vi "api_mqttSubscribe.vi"(0 "mqtt.lvclass in":refnum<class "mqtt.lvclass">, 5 "subscriptionInfo":T1[](array[typedef])=[{"Topic"="a/b", "QoS"=enum."At least once"}], 9 "messageID":u16=1, 11 "error in (no error)":errorcluster) -> (4 "mqtt.lvclass out":refnum<class "mqtt.lvclass">, 6 "success":bool, 15 "error out":errorcluster)   [LabVIEW 2018, in "labview-mqtt.lvlib" / "mqtt.lvclass"]
uses:
  mqtt.lvclass
  mqttTypedef/mqttSubscribeCluster.ctl
  mqttTypedef/mqttQOSlevel.ctl
  mqttTypedef/mqttMessageType.ctl
  mqttCmd/mqttCmdSubscribe/mqttCmdSubscribe.lvclass
  D:/mqtt-LabVIEW/src/class/mqtt/mqttCmd/mqttCmd.lvclass
  mqttCmd/mqttCmdSubscribe/mqttCmdSubscribe.lvclass/mqttCmdSubscribe.ctl
  mqttCmd/mqttCmd.lvclass/mqttCmd.ctl
  mqttCmd/mqttCmd.lvclass
  labview-mqtt.lvlib
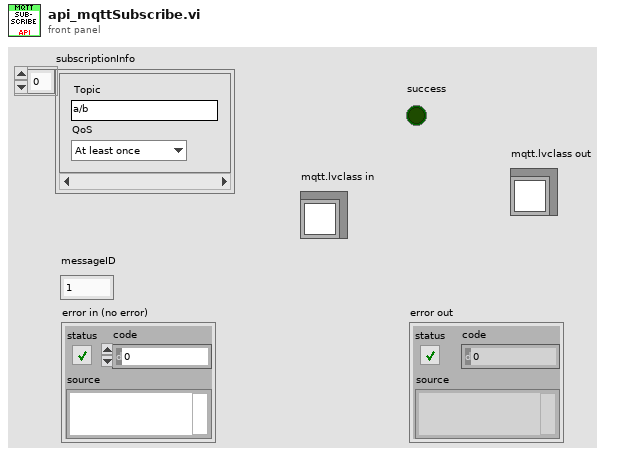
[diagram p1: front panel]
types:
  T1 = typedef "labview-mqtt.lvlib/mqttSubscribeCluster.ctl" = cluster{"Topic":string, "QoS":T2}
  T2 = typedef "labview-mqtt.lvlib/mqttQOSlevel.ctl" = enum8{"At most once", "At least once", "Exactly once", "Reserved"}
  T3 = typedef "labview-mqtt.lvlib/mqttMessageType.ctl" = enum32{"Reserved", "CONNECT", "CONNACK", "PUBLISH", "PUBACK", "PUBREC", "PUBREL", "PUBCOMP", "SUBSCRIBE", "SUBACK", "UNSUBSCRIBE", "UNSUBACK", "PINGREQ", "PINGRESP", "DISCONNECT", "Reserved2"}
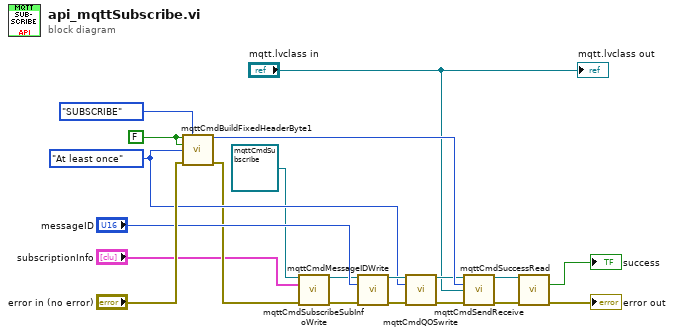
[diagram p0: block diagram]
diagram:
  w8 = mqttQOSlevel."At least once" ("QoS (At most once)")
  w2 = FALSE ("retain(F)")
  n1 = call "mqttCmdBuildFixedHeaderByte1.vi"("retain(F)"=w2, "MessageType"=mqttMessageType."SUBSCRIBE", "duplicate(F)"=w2, "QoS (At most once)"=w8, "error in (no error)"="error in (no error)") -> ("byte1"=w19:u8, "error out"=w7:errorcluster)  [unwired: 9 in]
  n2 = call "mqttCmdSubscribeSubInfoWrite.vi"("mqttSubscribe in"=refnum<class "mqttCmdSubscribe.lvclass"> refnum ("mqttSubscribe.lvclass"), "subscriptionInfo"="subscriptionInfo", "error in (no error)"=w7) -> ("mqttSubscribe out"=w5:refnum<class "mqttCmdSubscribe.lvclass">, "error out"=w6:errorcluster)  [unwired: 11 in]
  n3 = call "mqttCmdMessageIDWrite.vi"("mqttBrokerCommand in"=w5, "messageID"="messageID", "error in (no error)"=w6) -> ("mqttBrokerCommand out"=w10:refnum<class "mqttCmdSubscribe.lvclass">, "error out"=w12:errorcluster)  [unwired: 11 in]
  n4 = call "mqttCmdQOSwrite.vi"("mqttBrokerCommand in"=w10, "QoS"=w8, "error in (no error)"=w12) -> ("mqttBrokerCommand out"=w9:refnum<class "mqttCmdSubscribe.lvclass">, "error out"=w11:errorcluster)  [unwired: 11 in]
  n5 = call "mqttCmdSendReceive.vi"("mqttConnect in"=w9, "byte1"=w19, "mqtt in"="mqtt.lvclass in", "error in (no error)"=w11) -> ("mqttConnect out"=w16:refnum<class "mqttCmdSubscribe.lvclass">, "error out"=w17:errorcluster)  [unwired: 9 in, 1 out]
  n6 = call "mqttCmdSuccessRead.vi"("mqttBrokerCommand in"=w16, "error in (no error)"=w17) -> ("success"=→"success":bool, "error out"=→"error out":errorcluster)  [unwired: 11 in, 1 out]
  "mqtt.lvclass out" <- "mqtt.lvclass in"
